vi "UHR-Fleezers Control (host) - 11.8.vi"() -> ()   [LabVIEW 2014] (continued)
        n1567 = local write "Trap Pos. FB Offset Factor"(w2207) -> ()
      }
      event "Trap Pos. FB Range", "Trap Pos. FB Gains", "Trap Pos. FB Mult Factor", "Trap Pos. FB Offset Factor", "Trap Pos FB Negate Action", "Trap Pos FB Monitor\nT1 or T2", "Differential FB?", "Negate Diff?": Value Change {
        n1568 = event-data() -> ()  [unwired: 7 out]
        n1569 = local read "Negate Diff?"() -> (w2221:bool)
        n1570 = xnode "Read/Write Control"("FPGA VI Reference In"=w2231, "error in"=w2230, "Trap Pos. FB Range"="Trap Pos. FB Range", "Trap Pos. FB Gains"="Trap Pos. FB Gains", "Trap Pos. FB Mult Factor"="Trap Pos. FB Mult Factor", "Trap Pos. FB Offset Factor"="Trap Pos. FB Offset Factor", "Trap Pos FB Negate Action"="Trap Pos FB Negate Action", "Trap Pos FB Monitor T1 or T2"="Trap Pos FB Monitor\nT1 or T2", "AI1 X Scale"="Trap Pos. AI1 X Pre-scale", "Negate Diff?"=w2221, "Diff FB Measurement?"="Differential FB?") -> ()  [unwired: 2 out]
      }
      event "Trap Pos FB SP", "Trap Pos FB SP 2", "Use SP 2": Value Change {
        n1571 = event-data() -> ()  [unwired: 7 out]
        n1572 = Select(t="Trap Pos FB SP 2", s="Use SP 2", f="Trap Pos FB SP") -> (s? t:f=w2232:fxp<+/-,16,1>)
        n1573 = xnode "Read/Write Control"("FPGA VI Reference In"=w2237, "error in"=w2236, "Trap Pos. FB SP"=w2232) -> ()  [unwired: 2 out]
      }
      event "Offset SP2 from SP1": Value Change {
        n1574 = event-data() -> ()  [unwired: 7 out]
        n1575 = local read "Trap Pos FB SP"() -> (w2240:fxp<+/-,16,1>)
        n1576 = Add(x=w2240, y="SP2 Offset") -> (x+y=w2238:fxp<+/-,16,1>)
        n1577 = property on="Trap Pos FB SP 2" class="DigNum (strict)"("Val(Sgnl)"=w2238) -> ()  [unwired: 2 in, 2 out]
        n1578 = local write "Offset SP2 from SP1"(FALSE ("Offset SP2 from SP1")) -> ()
      }
      event "Set Reading to\nSetpoint": Value Change {
        # "This is the actual PID input signal"
        n1579 = event-data() -> ()  [unwired: 7 out]
        n1580 = local write "Set Reading to\nSetpoint"(FALSE ("Set SP to Reading")) -> ()
        n1581 = xnode "Read/Write Control"("FPGA VI Reference In"=w2246, "error in"=w2245) -> ("FPGA VI Reference Out"=w2244:T19, "error out"=w2243:errorcluster, "Trap Pos FB Int-Norm Signal"=w2242:fxp<+/-,16,1>)
        n1582 = local read "Differential FB?"() -> (w2247:bool)
        n1583 = case shown="False" w2247 {
          tunnel: [w2252 w2259] -> w2249
          tunnel: w2242 -> [w2250 w2259]
          frame False {
            n1584 = local read "Trap Pos FB Monitor\nT1 or T2"() -> (w2255:bool)
            n1585 = local read "Trap X AI1 (DMA)"() -> (w2258:T13)
            n1586 = Unbundle By Name(w2258) -> ("Set 1"=w2257:fxp<+/-,16,1>, "Set 2"=w2256:fxp<+/-,16,1>)
            n1587 = Select(t=w2257, s=w2255, f=w2256) -> (s? t:f=w2254:fxp<+/-,16,1>)
            n1588 = Not(x="Set SP Using...") -> (.not. x?=w2251:bool)
            n1589 = Select(t=w2250, s=w2251, f=w2254) -> (s? t:f=w2252:fxp<+/-,16,1>)
          }
          frame True {
          }
        }
        n1590 = xnode "Read/Write Control"("FPGA VI Reference In"=w2244, "error in"=w2243, "Trap Pos. FB SP"=w2249) -> ()  [unwired: 2 out]
        n1591 = local write "Trap Pos FB SP"(w2249) -> ()
      }
      event "Trap Pos. FB Out Scale 2^n": Value Change {
        n1592 = event-data() -> ()  [unwired: 7 out]
        n1593 = Scale By Power Of 2(n="Trap Pos. FB Out Scale 2^n", x=ext 1.0) -> (x*2^n=w2260:ext)
        n1594 = property on="Trap Pos. FB Mult Factor" class="DigNum (strict)"("Val(Sgnl)"=w2260) -> ()  [unwired: 2 in, 2 out]
      }
      event "Trap Pos FB Int Count": Value Change {
        n1595 = event-data() -> ()  [unwired: 7 out]
        n1596 = xnode "Read/Write Control"("FPGA VI Reference In"=w2265, "error in"=w2264, "Trap Pos FB Int Count"="Trap Pos FB Int Count") -> ()  [unwired: 2 out]
      }
      event "Trap pos": Value Change {
        n1597 = event-data() -> ()  [unwired: 7 out]
        n1598 = case shown="True" "Trap pos" {
          frame False {
            n1599 = property on="Trap Delta Graph" class="WFGraph (strict)"("Visible"=TRUE) -> ()  [unwired: 2 in, 2 out]
            n1600 = property on="Saved trap pos" class="WFGraph (strict)"("Visible"=FALSE) -> ()  [unwired: 2 in, 2 out]
          }
          frame True {
            n1601 = property on="Saved trap pos" class="WFGraph (strict)"("Visible"=TRUE) -> ()  [unwired: 2 in, 2 out]
            n1602 = property on="Trap Delta Graph" class="WFGraph (strict)"("Visible"=FALSE) -> ()  [unwired: 2 in, 2 out]
          }
        }
      }
      event "Save user params": Value Change {
        n1603 = event-data() -> ()  [unwired: 7 out]
        n1604 = local write "Save user params"(FALSE ("Save user\nparams")) -> ()
        n1605 = call "save control values.vi"("User"="User") -> ()  [unwired: 8 in, 1 out]
        n1606 = local read "Messages"() -> (w2277:string)
        n1607 = Concatenate Strings("User: ", "User", "\r", "Parameters saved.") -> (w2272:string)
        n1608 = call "Update messages.vi"("Message to add"=w2272, "Old message string"=w2277) -> ("New message string"=w2271:string)
        n1609 = local write "Messages"(w2271) -> ()
      }
      event "Load user params": Value Change {
        n1610 = event-data() -> ()  [unwired: 7 out]
        n1611 = local write "Load user params"(FALSE ("Read user\nparams")) -> ()
        n1612 = flat-sequence {
          tunnel: [w2309] -> w2297
          tunnel: [w2308] -> w2295
          tunnel: [w2307] -> w2293
          tunnel: [w2306] -> w2291
          tunnel: [w2305] -> w2289
          tunnel: [w2304] -> w2287
          tunnel: [w2303] -> w2285
          tunnel: [w2302] -> w2283
          tunnel: [w2301] -> w2281
          tunnel: [w2300] -> w2279
          tunnel: [w2319] -> w2298
          tunnel: w2297 -> [w2319]
          tunnel: [w2318] -> w2296
          tunnel: w2295 -> [w2318]
          tunnel: [w2317] -> w2294
          tunnel: w2293 -> [w2317]
          tunnel: [w2316] -> w2292
          tunnel: w2291 -> [w2316]
          tunnel: [w2315] -> w2290
          tunnel: w2289 -> [w2315]
          tunnel: [w2314] -> w2288
          tunnel: w2287 -> [w2314]
          tunnel: [w2313] -> w2286
          tunnel: w2285 -> [w2313]
          tunnel: [w2312] -> w2284
          tunnel: w2283 -> [w2312]
          tunnel: [w2311] -> w2282
          tunnel: w2281 -> [w2311]
          tunnel: [w2310] -> w2280
          tunnel: w2279 -> [w2310]
          tunnel: w2298 -> [w2336]
          tunnel: w2296 -> [w2335]
          tunnel: w2294 -> [w2334]
          tunnel: w2292 -> [w2333]
          tunnel: w2290 -> [w2332]
          tunnel: w2288 -> [w2331]
          tunnel: w2286 -> [w2330]
          tunnel: w2284 -> [w2329]
          tunnel: w2282 -> [w2328]
          tunnel: w2280 -> [w2327]
          frame #0 {
            # "Make exceptions.\nThese will not be\nloaded."
            n1613 = local read "Green Laser ON/Interlacing"() -> (w2305:bool)
            n1614 = local read "Sample Channel\nFlow"() -> (w2304:bool)
            n1615 = local read "Trap 1 (ON/OFF)"() -> (w2309:bool)
            n1616 = local read "Trap 2 (ON/OFF)"() -> (w2308:bool)
            n1617 = local read "Trap Pos. FB ON"() -> (w2300:bool)
            n1618 = local read "Inject Pump 1"() -> (w2303:bool)
            n1619 = local read "Inject Pump 3"() -> (w2302:bool)
            n1620 = local read "Trap D (MHz)"() -> (w2301:dbl)
            n1621 = local read "Index"() -> (w2306:dbl)
            n1622 = local read "Fish"() -> (w2307:bool)
          }
          frame #1 {
            n1623 = local read "User"() -> (w2320:string)
            n1624 = call "retrieve control values.vi"("User"=w2320) -> ()  [unwired: 10 in, 1 out]
            n1625 = local read "Messages"() -> (w2326:string)
            n1626 = Concatenate Strings("User: ", w2320, "\r", "Parameters loaded.") -> (w2321:string)
            n1627 = call "Update messages.vi"("Message to add"=w2321, "Old message string"=w2326) -> ("New message string"=w2325:string)
            n1628 = local write "Messages"(w2325) -> ()
          }
          frame #2 {
            n1629 = local write "Green Laser ON/Interlacing"(w2332) -> ()
            n1630 = local write "Sample Channel\nFlow"(w2331) -> ()
            n1631 = local write "Trap 1 (ON/OFF)"(w2336) -> ()
            n1632 = local write "Trap 2 (ON/OFF)"(w2335) -> ()
            n1633 = local write "Inject Pump 1"(w2330) -> ()
            n1634 = local write "Trap Pos. FB ON"(w2327) -> ()
            n1635 = local write "Inject Pump 3"(w2329) -> ()
            n1636 = local write "Trap D (MHz)"(w2328) -> ()
            n1637 = local write "Index"(w2333) -> ()
            n1638 = local write "Fish"(w2334) -> ()
          }
        }
      }
      event "Abort wiggle": Value Change {
        n1639 = event-data() -> ()  [unwired: 7 out]
        n1640 = flat-sequence {
          tunnel: w2340 -> [w2344]
          tunnel: w2339 -> [w2343]
          tunnel: [w2342] -> w2337
          tunnel: [w2346] -> w2338
          tunnel: w2337 -> [w2346]
          frame #0 {
            n1641 = xnode "Read/Write Control"("FPGA VI Reference In"=w2344, "error in"=w2343, "Abort wiggle 1"="Abort wiggle", "Abort wiggle 2"="Abort wiggle") -> ("error out"=w2342:errorcluster)  [unwired: 1 out]
          }
          frame #1 {
            n1642 = local write "Abort wiggle"(FALSE ("Abort wiggle")) -> ()
          }
        }
      }
    }
    "error out 2" <- w1142
    n1643 = node-c288() -> ()  [unwired: 2 out]
  }
  n1644 = node-c288() -> (w96:T21)  [unwired: 4 in]
  n1645 = node-c288() -> (w110:T21)  [unwired: 4 out]
  n1646 = timed-loop "Run Scripts, including: stage motion" {
    tunnel: w101 -> [w2354]
    tunnel: w100 -> [w2355]
    tunnel: [w2355] -> w99
    tunnel: [w2354] -> w98
    timing: w96 -> [_]
    timing-out: [_] -> w95
    tunnel: w81 -> [w2353]
    tunnel: w82 -> [w2352]
    tunnel: w22 -> [w2349]
    tunnel: w21 -> [w2348]
    tunnel: w20 -> [w2350]
    tunnel: w19 -> [w2351]
    stop <- w2347 stop-if-true
    n1647 = node-c288() -> ()  [unwired: 1 in, 1 out]
    n1648 = event shown="[12] \"Force FB Script\": Value Change" {
      selector: _ -> [_ _ _ _ _ _ _ _ _ _ _ _ _ _ _ _ _ _ _ _]
      dyn-events: _ -> [_ _ _ _ _ _ _ _ _ _ _ _ _ _ _ _ _ _ _ _]
      timeout: _ -> [_ _ _ _ _ _ _ _ _ _ _ _ _ _ _ _ _ _ _ _]
      tunnel: ["Set Position" "Move to Position" _ _ "Read Harvard" _ _ _ _ _ _ "Got ADig bead" "Force FB Script" "Rupture Script" _ "Got DNA bead" "Take Stepping Data" _ "Take Detection Laser\nImage" _] -> _
      tunnel: [_ _ _ _ _ _ _ _ _ _ _ _ _ _ _ _ _ _ _ w3010] -> w2347
      tunnel: w2354 -> [w2373 w2381 w2394 w2424 _ w2471 w2511 w2592 w2623 w2757 w2783 _ w2821 _ _ _ _ _ _ _]
      tunnel: w2355 -> [w2374 w2382 w2395 w2425 _ w2472 w2512 w2593 w2624 w2758 w2784 _ w2822 _ _ _ _ _ _ _]
      tunnel: w2353 -> [_ _ _ _ w2456 _ _ _ _ _ _ _ _ _ _ _ _ _ _ _]
      tunnel: w2352 -> [_ _ _ _ w2455 _ _ _ _ _ _ _ _ _ _ _ _ _ _ _]
      tunnel: w2351 -> [_ _ _ _ _ _ _ _ _ _ _ _ _ _ _ _ _ _ _ _]
      tunnel: w2350 -> [_ _ _ _ _ _ _ _ _ _ _ _ _ _ _ _ _ _ _ _]
      tunnel: w2349 -> [_ _ _ _ _ _ _ _ _ _ _ _ _ _ _ _ _ _ _ _]
      tunnel: w2348 -> [_ _ _ _ _ _ _ _ _ _ _ _ _ _ _ _ _ _ _ _]
      event "Set Position", "Set Position 2", "Set Position 3", "Set Position 4", "Set Position 5", "Set Position 1": Value Change {
        n1649 = event-data() -> ()  [unwired: 1 in, 5 out]
        n1650 = Build Array("Set Position 1", "Set Position 2", "Set Position 3", "Set Position 4", "Set Position 5") -> (w2372:bool[])
        n1651 = Boolean Array To Number(Boolean array=w2372) -> (number=w2371:u32)
        n1652 = Logarithm Base 2(1:w2371) -> (0:w2363:dbl)
        n1653 = call "Read Stage Position.vi"("error in"=w2373, "VISA resource name in"=w2374) -> ("Current Position"=w2378:cluster{dbl, dbl, dbl}, "error out"=w2377:errorcluster)  [unwired: 2 out]
        n1654 = Decrement(x="Position") -> (x-1=w2361:dbl)
        n1655 = Greater Or Equal?(x=w2363, y=0.0) -> (x >= y?=w2364:bool)
        n1656 = Cluster To Array(cluster=w2378) -> (array=w2375:dbl[])
        n1657 = local write "Stage Control Serial Error"(w2377) -> ()
        n1658 = Select(t=w2363, s=w2364, f=w2361) -> (s? t:f=w2360:dbl)
        n1659 = Increment(x=w2360) -> (x+1=w2359:dbl)
        n1660 = Build Array (concatenate)(w2359, w2375) -> (w2358:dbl[])
        n1661 = Replace Array Subset(array="Saved Stage Positions", new element=w2358, index (row)=w2360) -> (w2376:dbl[][])  [unwired: 1 in]
        n1662 = local write "Saved Stage Positions"(w2376) -> ()
      }
      event "Move to Position": Value Change {
        n1663 = event-data() -> ()  [unwired: 1 in, 5 out]
        n1664 = flat-sequence {
          tunnel: w2382 -> [w2386]
          tunnel: w2381 -> [w2385]
          frame #0 {
            n1665 = local read "Saved Stage Positions"() -> (w2388:dbl[][])
            n1666 = local read "Position"() -> (w2387:dbl)
            n1667 = local write "Stage Moving"(TRUE ("Stage Moving")) -> ()
            n1668 = call "move to saved stage position.vi"("error in"=w2385, "Stage VISA resource name in"=w2386, "Position"=w2387, "Saved Stage Positions"=w2388) -> ("error out"=w2384:errorcluster)  [unwired: 1 out]
            n1669 = local write "Stage Control Serial Error"(w2384) -> ()
          }
          frame #1 {
            n1670 = call <vilib>:"Beep.vi"() -> ()  [unwired: 3 in, 9 out]
            n1671 = local write "Stage Moving"(FALSE ("Stage Moving")) -> ()
          }
        }
      }
      event "Move Cap. 1 (DNA Bottom)": Value Change {
        n1672 = event-data() -> ()  [unwired: 1 in, 5 out]
        n1673 = local write "Move Cap. 1 (DNA Bottom)"(FALSE ("Move Cap. 1 (DNA Right)")) -> ()
        n1674 = flat-sequence {
          tunnel: w2394 -> [w2397]
          tunnel: w2395 -> [w2398]
          tunnel: [w2398] -> w2392
          tunnel: [w2397] -> w2391
          tunnel: w2392 -> [w2400]
          tunnel: w2391 -> [w2399]
          frame #0 {
            n1675 = property on="Sample Channel\nFlow" class="Bool (strict)"("Val(Sgnl)"="Cap 1 Samp Flow ON") -> ()  [unwired: 2 in, 2 out]
          }
          frame #1 {
            n1676 = local read "Saved Stage Positions"() -> (w2410:dbl[][])
            n1677 = local write "Stage Moving"(TRUE ("Stage Moving")) -> ()
            n1678 = Array Subset(array=w2410, index (row)=0 ("index"), length (row)=1 ("length"), index (col)=1 ("index"), length (col)=3 ("length")) -> (w2407:dbl[][])
            n1679 = Reshape Array(w2407, 3 ("dimension size")) -> (w2405:dbl[])
            n1680 = Array To Cluster(array=w2405) -> (cluster=w2404:cluster{"[0]":dbl, "[1]":dbl, "[2]":dbl})
            n1681 = call "Set Stage Position.vi"("Position"=w2404, "error in"=w2399, "VISA resource name in"=w2400) -> ("error out"=w2403:errorcluster)  [unwired: 2 out]
            n1682 = local write "Stage Control Serial Error"(w2403) -> ()
          }
          frame #2 {
            n1683 = local write "Stage Moving"(FALSE ("Stage Moving")) -> ()
            n1684 = case shown="True" "Cap 1 Flow ON" {
              frame False {
              }
              frame True {
                n1685 = property on="Inject Pump 1" class="Bool (strict)"("Val(Sgnl)"=TRUE ("Value (Signaling)")) -> ()  [unwired: 2 in, 2 out]
              }
            }
            n1686 = call <vilib>:"Beep.vi"() -> ()  [unwired: 3 in, 9 out]
          }
          frame #3 {
            n1687 = property on="Sample Channel\nFlow" class="Bool (strict)"("Val(Sgnl)"=FALSE ("Value (Signaling)")) -> ()  [unwired: 2 in, 2 out]
            n1688 = local read "Cap. 2 BD T1?\n(ADig T1, DNA T2)"() -> (w2417:bool)
            n1689 = case shown="True" w2417 {
              tunnel: "Cap 1 T ON" -> [w2419 w2420]
              frame False {
                n1690 = property on="Trap 1 (ON/OFF)" class="Bool (strict)"("Val(Sgnl)"=w2419) -> ()  [unwired: 2 in, 2 out]
              }
              frame True {
                n1691 = property on="Trap 2 (ON/OFF)" class="Bool (strict)"("Val(Sgnl)"=w2420) -> ()  [unwired: 2 in, 2 out]
              }
            }
            n1692 = property on="Got DNA bead" class="Bool"("Key Focus"=TRUE) -> ()  [unwired: 2 in, 2 out]
          }
        }
      }
      event "Move Cap. 2 (ADig Top)": Value Change {
        n1693 = event-data() -> ()  [unwired: 1 in, 5 out]
        n1694 = local write "Move Cap. 2 (ADig Top)"(FALSE ("Move Cap. 2 (ADig Left)")) -> ()
        n1695 = flat-sequence {
          tunnel: w2424 -> [w2427]
          tunnel: w2425 -> [w2428]
          tunnel: [w2428] -> w2422
          tunnel: [w2427] -> w2421
          tunnel: w2422 -> [w2431]
          tunnel: w2421 -> [w2430]
          frame #0 {
            n1696 = property on="Sample Channel\nFlow" class="Bool (strict)"("Val(Sgnl)"="Cap 2 Samp Flow ON") -> ()  [unwired: 2 in, 2 out]
          }
          frame #1 {
            w2429 = FALSE ("Value (Signaling)")
            n1697 = local read "Saved Stage Positions"() -> (w2441:dbl[][])
            n1698 = local write "Stage Moving"(TRUE ("Stage Moving")) -> ()
            n1699 = Array Subset(array=w2441, index (row)=1 ("index"), length (row)=1 ("length"), index (col)=1 ("index"), length (col)=3 ("length")) -> (w2438:dbl[][])
            n1700 = Reshape Array(w2438, 3 ("dimension size")) -> (w2436:dbl[])
            n1701 = property on="Trap 1 (ON/OFF)" class="Bool (strict)"("Val(Sgnl)"=w2429) -> ()  [unwired: 2 in, 2 out]
            n1702 = property on="Trap 1 (ON/OFF)" class="Bool (strict)"("Val(Sgnl)"=w2429) -> ()  [unwired: 2 in, 2 out]
            n1703 = Array To Cluster(array=w2436) -> (cluster=w2435:cluster{"[0]":dbl, "[1]":dbl, "[2]":dbl})
            n1704 = call "Set Stage Position.vi"("Position"=w2435, "error in"=w2430, "VISA resource name in"=w2431) -> ("error out"=w2434:errorcluster)  [unwired: 2 out]
            n1705 = local write "Stage Control Serial Error"(w2434) -> ()
          }
          frame #2 {
            n1706 = local write "Stage Moving"(FALSE ("Stage Moving")) -> ()
            n1707 = call <vilib>:"Beep.vi"() -> ()  [unwired: 3 in, 9 out]
            n1708 = case shown="True" "Cap 2 Flow ON" {
              frame False {
              }
              frame True {
                n1709 = property on="Inject Pump 3" class="Bool (strict)"("Val(Sgnl)"=TRUE ("Value (Signaling)")) -> ()  [unwired: 2 in, 2 out]
              }
            }
          }
          frame #3 {
            n1710 = local read "Cal @ (MHz)"() -> (w2447:dbl)
            n1711 = property on="Sample Channel\nFlow" class="Bool (strict)"("Val(Sgnl)"=FALSE ("Value (Signaling)")) -> ()  [unwired: 2 in, 2 out]
            n1712 = case shown="False" "Cap. 2 BD T1?\n(ADig T1, DNA T2)" {
              tunnel: "Cap 2 T ON" -> [w2452 w2453]
              frame False {
                n1713 = property on="Trap 2 (ON/OFF)" class="Bool (strict)"("Val(Sgnl)"=w2452) -> ()  [unwired: 2 in, 2 out]
              }
              frame True {
                n1714 = property on="Trap 1 (ON/OFF)" class="Bool (strict)"("Val(Sgnl)"=w2453) -> ()  [unwired: 2 in, 2 out]
              }
            }
            n1715 = property on="Got ADig bead" class="Bool"("Key Focus"=TRUE) -> ()  [unwired: 2 in, 2 out]
            n1716 = local write "Target"("Target\nON?") -> ()
            n1717 = property on="Trap D (MHz)" class="DigNum (strict)"("Val(Sgnl)"=w2447) -> ()  [unwired: 2 in, 2 out]
          }
        }
      }
      event "Read Harvard": Value Change {
        n1718 = event-data() -> ()  [unwired: 1 in, 5 out]
        n1719 = Concatenate Strings("write buffer", "\r") -> (w2458:string)
        n1720 = VISA Write(VISA resource name=w2456, write buffer=w2458, error in (no error)=w2455) -> (VISA resource name out=w2467:refnum<visa-resource-name>, error out=w2466:errorcluster)  [unwired: 1 out]
        n1721 = stacked-sequence {
          tunnel: [w2470] -> w2465
          tunnel: w2467 -> [w2470]
          tunnel: w2466 -> [w2469]
          tunnel: [w2469] -> w2460
          frame #0 {
            n1722 = Wait (ms)(milliseconds to wait=50) -> ()  [unwired: 1 out]
          }
        }
        n1723 = property class="Instr"(reference=w2465, error in=w2460) -> (reference out=w2464:refnum<visa-resource-name>, error out=w2462:errorcluster, "Serial Settings:Number of Bytes at Serial Port"=w2463:u32)
        "Serial Settings:Number of Bytes at Serial Port" <- w2463
        n1724 = VISA Read(VISA resource name=w2464, byte count=w2463, error in (no error)=w2462) -> (read buffer=w2461:string)  [unwired: 3 out]
        "read buffer" <- w2461
        n1725 = Fract/Exp String To Number(string=w2461) -> ()  [unwired: 5 out]
      }
      event "+z", "-z": Value Change {
        n1726 = event-data() -> ()  [unwired: 1 in, 5 out]
        n1727 = flat-sequence {
          tunnel: w2471 -> [w2493]
          tunnel: w2472 -> [w2473]
          frame #0 {
            n1728 = call "Read Stage Position.vi"("error in"=w2493, "VISA resource name in"=w2473) -> ("Current Position"=w2478:cluster{dbl, dbl, dbl}, "error out"=w2491:errorcluster, "VISA resource name out"=w2492:refnum<visa-resource-name>)  [unwired: 1 out]
            n1729 = local read "Saved Stage Positions"() -> (w2502:dbl[][])
            n1730 = Divide(x="z nudge increment (um)", y=1000.0) -> (x/y=w2490:dbl)
            n1731 = Boolean To (0,1)(Boolean="+z") -> (0, 1=w2482:i16)
            n1732 = Boolean To (0,1)(Boolean="-z") -> (0, 1=w2483:i16)
            n1733 = Array Subset(array=w2502, index (row)=1 ("index"), length (row)=1 ("length"), index (col)=1 ("index"), length (col)=3 ("length")) -> (w2499:dbl[][])
            n1734 = Multiply(x=w2482, y=w2490) -> (x*y=w2486:dbl)
            n1735 = Multiply(x=w2483, y=w2490) -> (x*y=w2484:dbl)
            n1736 = Unbundle(w2478) -> (w2476:dbl, w2475:dbl, w2479:dbl)
            n1737 = Negate(x=w2484) -> (-x=w2485:dbl)
            n1738 = Reshape Array(w2499, 3 ("dimension size")) -> (w2497:dbl[])
            n1739 = Add(x=w2486, y=w2485) -> (x+y=w2487:dbl)
            n1740 = Array To Cluster(array=w2497) -> ()  [unwired: 1 out]
            n1741 = Add(x=w2487, y=w2479) -> (x+y=w2477:dbl)
            n1742 = Bundle(cluster=w2478, w2476, w2475, w2477) -> (w2474:cluster{dbl, dbl, dbl})
            n1743 = call "Set Stage Position.vi"("Position"=w2474, "error in"=w2491, "VISA resource name in"=w2492) -> ("error out"=w2496:errorcluster)  [unwired: 2 out]
            n1744 = local write "Stage Moving"(TRUE ("Stage Moving")) -> ()
            n1745 = local write "Stage Control Serial Error"(w2496) -> ()
          }
          frame #1 {
            n1746 = local write "Stage Moving"(FALSE ("Stage Moving")) -> ()
            n1747 = call <vilib>:"Beep.vi"() -> ()  [unwired: 3 in, 9 out]
          }
        }
      }
      event "Cal/Data Acq. Spot": Value Change {
        n1748 = event-data() -> ()  [unwired: 1 in, 5 out]
        n1749 = flat-sequence {
          tunnel: w2511 -> [w2515]
          tunnel: w2512 -> [w2516]
          tunnel: [w2516] -> w2508
          tunnel: [w2515] -> w2507
          tunnel: w2508 -> [w2521]
          tunnel: w2507 -> [w2520]
          tunnel: ["Cal @ (MHz)"] -> w2505
          tunnel: [w2525] -> w2509
          tunnel: w2505 -> [w2525]
          tunnel: w2509 -> [w2534]
          tunnel: ["W/ Offset 1"] -> w2506
          tunnel: w2509 -> [w2555]
          tunnel: w2506 -> [w2553]
          frame #0 {
            n1750 = property on="Sample Channel\nFlow" class="Bool (strict)"("Val(Sgnl)"="Daq spot flow on") -> ()  [unwired: 2 in, 2 out]
            n1751 = Wait (ms)(milliseconds to wait=u32 250) -> ()  [unwired: 1 out]
          }
          frame #1 {
            n1752 = local read "Saved Stage Positions"() -> (w2518:dbl[][])
            n1753 = property on="Trap D (MHz)" class="DigNum (strict)"("Val(Sgnl)"="Cal @ (MHz)") -> ()  [unwired: 2 in, 2 out]
            n1754 = local write "Stage Moving"(TRUE ("Stage Moving")) -> ()
            n1755 = call "move to saved stage position.vi"("error in"=w2520, "Stage VISA resource name in"=w2521, "Position"="Cal Stage Position", "Saved Stage Positions"=w2518) -> ("error out"=w2519:errorcluster)  [unwired: 1 out]
            n1756 = local write "Stage Control Serial Error"(w2519) -> ()
          }
          frame #2 {
            n1757 = local write "Stage Moving"(FALSE ("Stage Moving")) -> ()
            n1758 = property on="Sample Channel\nFlow" class="Bool (strict)"("Val(Sgnl)"="Flow ON\nduring cal?") -> ()  [unwired: 2 in, 2 out]
            n1759 = call <vilib>:"Beep.vi"() -> ()  [unwired: 3 in, 9 out]
          }
          frame #3 {
            n1760 = Wait (ms)(milliseconds to wait=u32 1000) -> ()  [unwired: 1 out]
          }
          frame #4 {
            n1761 = property on="Save Calibration" class="Bool (strict)"("Val(Sgnl)"=TRUE ("Value (Signaling)")) -> ()  [unwired: 2 in, 2 out]
          }
          frame #5 {
            n1762 = Wait (ms)(milliseconds to wait=u32 2000) -> ()  [unwired: 1 out]
          }
          frame #6 {
            # "Check to see if \nsaving done"
            n1763 = while {
              stop <- w2530 stop-if-true
              n1764 = local read "Saving..."() -> (w2531:bool)
              n1765 = Wait (ms)(milliseconds to wait=u32 100) -> ()  [unwired: 1 out]
              n1766 = Not(x=w2531) -> (.not. x?=w2530:bool)
            }
          }
          frame #7 {
            n1767 = case shown="True" "W/ Offset 1" {
              tunnel: w2534 -> [_ w2535]
              frame False {
              }
              frame True {
                n1768 = stacked-sequence {
                  tunnel: w2535 -> [_ _ _ _ _ _ _ w2552]
                  frame #0 {
                    n1769 = property on="Trap D (MHz)" class="DigNum (strict)"("Val(Sgnl)"="Offset 1 Start (MHz)") -> ()  [unwired: 2 in, 2 out]
                    n1770 = Replace Array Subset(array=u32[] [0] ("Index Values"), new element="Offset 1 Set", index=0) -> (w2536:u32[])
                    n1771 = property on="Saved AOD Raster Scan Parameter Sets" class="Arr (strict)"("Index Values"=w2536) -> ()  [unwired: 2 in, 2 out]
                  }
                  frame #1 {
                    n1772 = Wait (ms)(milliseconds to wait=u32 200) -> ()  [unwired: 1 out]
                  }
                  frame #2 {
                    n1773 = property on="Load parameters" class="Bool (strict)"("Val(Sgnl)"=TRUE ("Value (Signaling)")) -> ()  [unwired: 2 in, 2 out]
                  }
                  frame #3 {
                    n1774 = Wait (ms)(milliseconds to wait=u32 200) -> ()  [unwired: 1 out]
                  }
                  frame #4 {
                    n1775 = property on="Trap Raster Scan" class="Bool (strict)"("Val(Sgnl)"=TRUE ("Value (Signaling)")) -> ()  [unwired: 2 in, 2 out]
                  }
                  frame #5 {
                    n1776 = Wait (ms)(milliseconds to wait=u32 2000) -> ()  [unwired: 1 out]
                  }
                  frame #6 {
                    n1777 = while {
                      stop <- w2549 stop-if-true
                      n1778 = local read "Raster Scanning..."() -> (w2551:bool)
                      n1779 = local read "Saving..."() -> (w2547:bool)
                      n1780 = Wait (ms)(milliseconds to wait=u32 100) -> ()  [unwired: 1 out]
                      n1781 = Not(x=w2547) -> (.not. x?=w2546:bool)
                      n1782 = Not(x=w2551) -> (.not. x?=w2548:bool)
                      n1783 = And(x=w2548, y=w2546) -> (x .and. y?=w2549:bool)
                    }
                  }
                  frame #7 {
                    n1784 = property on="Trap D (MHz)" class="DigNum (strict)"("Val(Sgnl)"=w2552) -> ()  [unwired: 2 in, 2 out]
                  }
                }
              }
            }
          }
          frame #8 {
            n1785 = local read "Save ave N"() -> (w2554:dbl)
            n1786 = case shown="False" "W/ Offset 2" {
              tunnel: w2555 -> [_ w2562]
              tunnel: w2554 -> [_ w2561]
              tunnel: w2553 -> [w2557 _]
              frame False {
                n1787 = case shown="False" w2557 {
                  frame False {
                    n1788 = Multiply(x="Cal read wait (s)", y=u32 1000 ("milliseconds to wait")) -> (x*y=w2559:u32)
                    n1789 = Wait (ms)(milliseconds to wait=w2559) -> ()  [unwired: 1 out]
                  }
                  frame True {
                  }
                }
              }
              frame True {
                n1790 = stacked-sequence {
                  tunnel: w2562 -> [_ _ _ _ _ _ _ _ _ w2583 _ _]
                  tunnel: w2561 -> [_ _ _ _ _ _ _ _ _ w2581 _ _]
                  frame #0 {
                    n1791 = property on="Save ave N" class="DigNum (strict)"("Val(Sgnl)"=1.0 ("Value (Signaling)")) -> ()  [unwired: 2 in, 2 out]
                  }
                  frame #1 {
                    n1792 = Wait (ms)(milliseconds to wait=u32 500) -> ()  [unwired: 1 out]
                  }
                  frame #2 {
                    n1793 = property on="Trap D (MHz)" class="DigNum (strict)"("Val(Sgnl)"="Offset 2 Start (MHz)") -> ()  [unwired: 2 in, 2 out]
                    n1794 = Replace Array Subset(array=u32[] [0] ("Index Values"), new element="Offset 2 Set", index=0) -> (w2567:u32[])
                    n1795 = property on="Saved AOD Raster Scan Parameter Sets" class="Arr (strict)"("Index Values"=w2567) -> ()  [unwired: 2 in, 2 out]
                  }
                  frame #3 {
                    n1796 = Wait (ms)(milliseconds to wait=u32 500) -> ()  [unwired: 1 out]
                  }
                  frame #4 {
                    n1797 = property on="Load parameters" class="Bool (strict)"("Val(Sgnl)"=TRUE ("Value (Signaling)")) -> ()  [unwired: 2 in, 2 out]
                  }
                  frame #5 {
                    n1798 = Wait (ms)(milliseconds to wait=u32 500) -> ()  [unwired: 1 out]
                  }
                  frame #6 {
                    n1799 = property on="Trap Raster Scan" class="Bool (strict)"("Val(Sgnl)"=TRUE ("Value (Signaling)")) -> ()  [unwired: 2 in, 2 out]
                  }
                  frame #7 {
                    n1800 = Wait (ms)(milliseconds to wait=u32 2000) -> ()  [unwired: 1 out]
                  }
                  frame #8 {
                    n1801 = while {
                      stop <- w2576 stop-if-true
                      n1802 = local read "Raster Scanning..."() -> (w2579:bool)
                      n1803 = local read "Saving..."() -> (w2577:bool)
                      n1804 = Wait (ms)(milliseconds to wait=u32 100) -> ()  [unwired: 1 out]
                      n1805 = Not(x=w2577) -> (.not. x?=w2575:bool)
                      n1806 = Not(x=w2579) -> (.not. x?=w2578:bool)
                      n1807 = And(x=w2578, y=w2575) -> (x .and. y?=w2576:bool)
                    }
                  }
                  frame #9 {
                    n1808 = property on="Trap D (MHz)" class="DigNum (strict)"("Val(Sgnl)"=w2583) -> ()  [unwired: 2 in, 2 out]
                    n1809 = property on="Saved AOD Raster Scan Parameter Sets" class="Arr (strict)"("Index Values"=u32[] [0]) -> ()  [unwired: 2 in, 2 out]
                    n1810 = property on="Save ave N" class="DigNum (strict)"("Val(Sgnl)"=w2581) -> ()  [unwired: 2 in, 2 out]
                  }
                  frame #10 {
                    n1811 = Wait (ms)(milliseconds to wait=u32 500) -> ()  [unwired: 1 out]
                  }
                  frame #11 {
                    n1812 = property on="Load parameters" class="Bool (strict)"("Val(Sgnl)"=TRUE ("Value (Signaling)")) -> ()  [unwired: 2 in, 2 out]
                  }
                }
              }
            }
          }
          frame #9 {
            n1813 = property on="Read Cal" class="Bool (strict)"("Val(Sgnl)"=TRUE ("Value (Signaling)")) -> ()  [unwired: 2 in, 2 out]
          }
          frame #10 {
            n1814 = Wait (ms)(milliseconds to wait=u32 1000) -> ()  [unwired: 1 out]
          }
          frame #11 {
            n1815 = property on="Fish" class="Bool (strict)"("Val(Sgnl)"=TRUE ("Value (Signaling)")) -> ()  [unwired: 2 in, 2 out]
          }
        }
        n1816 = local write "Cal/Data Acq. Spot"(FALSE ("Cal/Data Acq. Spot")) -> ()
      }
      event "Dump Beads": Value Change {
        n1817 = event-data() -> ()  [unwired: 1 in, 5 out]
        n1818 = flat-sequence {
          tunnel: ["Dump spot flow on?"] -> w2589
          tunnel: [w2601] -> w2590
          tunnel: w2589 -> [w2601]
          tunnel: w2593 -> [w2606]
          tunnel: w2592 -> [w2605]
          tunnel: [w2603] -> w2591
          tunnel: w2590 -> [w2603]
          tunnel: w2591 -> [w2617]
          frame #0 {
            w2594 = FALSE ("Value (Signaling)")
            n1819 = local read "Saving..."() -> (w2596:bool)
            n1820 = local write "Dump Beads"(FALSE ("Dump Beads")) -> ()
            n1821 = property on="Inject Pump 3" class="Bool (strict)"("Val(Sgnl)"=w2594) -> ()  [unwired: 2 in, 2 out]
            n1822 = property on="Inject Pump 1" class="Bool (strict)"("Val(Sgnl)"=w2594) -> ()  [unwired: 2 in, 2 out]
            n1823 = local write "Stop Saving"(w2596) -> ()
            n1824 = local write "Fish"(w2594) -> ()
          }
          frame #1 {
            w2597 = TRUE
            w2598 = FALSE ("Fl. Triggered...")
            n1825 = case shown="True" "Dump spot flow on?" {
              frame False {
              }
              frame True {
                n1826 = property on="Sample Channel\nFlow" class="Bool (strict)"("Val(Sgnl)"=TRUE ("Stage Moving")) -> ()  [unwired: 2 in, 2 out]
              }
            }
            n1827 = local write "Fl. Triggered..."(w2598) -> ()
            n1828 = local write "Tether"(w2598) -> ()
            n1829 = local write "Multiple tether"(w2598) -> ()
            n1830 = local write "Good tether"(w2598) -> ()
            n1831 = property on="Green Laser ON/Interlacing" class="Bool (strict)"("Val(Sgnl)"=w2598) -> ()  [unwired: 2 in, 2 out]
            n1832 = property on="Trap Pos. FB ON" class="Bool (strict)"("Val(Sgnl)"=w2598) -> ()  [unwired: 2 in, 2 out]
            n1833 = property on="Trap Trig. Fl." class="Bool (strict)"("Val(Sgnl)"=w2598) -> ()  [unwired: 2 in, 2 out]
            n1834 = local write "Bad fit"(w2598) -> ()
            n1835 = local write "Hysteresis"(w2598) -> ()
            n1836 = property on="Fl. Triggered..." class="Bool (strict)"("Val(Sgnl)"=w2598) -> ()  [unwired: 2 in, 2 out]
            n1837 = local write "Restart DMA? (AOD)"(w2597) -> ()
            n1838 = local write "Save scans"(w2597) -> ()
            n1839 = property on="Dip for Protein" class="Bool (strict)"("Val(Sgnl)"=w2598) -> ()  [unwired: 2 in, 2 out]
            n1840 = property on="Pause dwell" class="Bool (strict)"("Val(Sgnl)"=w2598) -> ()  [unwired: 2 in, 2 out]
          }
          frame #2 {
            n1841 = property on="Trap Pos. FB Offset Factor" class="DigNum (strict)"("Val(Sgnl)"=i64 0 ("Value (Signaling)")) -> ()  [unwired: 2 in, 2 out]
          }
          frame #3 {
            n1842 = local read "Saved Stage Positions"() -> (w2607:dbl[][])
            n1843 = Array Subset(array=w2607, index (row)=3 ("index"), length (row)=1 ("length"), index (col)=1 ("index"), length (col)=3 ("length")) -> (w2612:dbl[][])
            n1844 = local write "Stage Moving"(TRUE ("Stage Moving")) -> ()
            n1845 = Reshape Array(w2612, 3 ("dimension size")) -> (w2610:dbl[])
            n1846 = Array To Cluster(array=w2610) -> (cluster=w2609:cluster{"[0]":dbl, "[1]":dbl, "[2]":dbl})
            n1847 = call "Set Stage Position.vi"("Position"=w2609, "error in"=w2605, "VISA resource name in"=w2606) -> ()  [unwired: 3 out]
          }
          frame #4 {
            w2618 = FALSE ("Value (Signaling)")
            n1848 = case shown="True" w2617 {
              frame False {
              }
              frame True {
                n1849 = property on="Sample Channel\nFlow" class="Bool (strict)"("Val(Sgnl)"=FALSE ("Stage Moving")) -> ()  [unwired: 2 in, 2 out]
              }
            }
            n1850 = property on="Trap 1 (ON/OFF)" class="Bool (strict)"("Val(Sgnl)"=w2618) -> ()  [unwired: 2 in, 2 out]
            n1851 = property on="Trap 2 (ON/OFF)" class="Bool (strict)"("Val(Sgnl)"=w2618) -> ()  [unwired: 2 in, 2 out]
            n1852 = call <vilib>:"Beep.vi"() -> ()  [unwired: 3 in, 9 out]
            n1853 = local write "Fish"(FALSE ("Fish for Tether")) -> ()
          }
          frame #5 {
            n1854 = property on="Move Cap. 2 (ADig Top)" class="Bool (strict)"("Val(Sgnl)"=TRUE ("Value (Signaling)")) -> ()  [unwired: 2 in, 2 out]
            n1855 = property on="Tab Control" class="TabCtl (strict)"("Val(Sgnl)"=T4."Status" ("Value (Signaling)")) -> ()  [unwired: 2 in, 2 out]
          }
        }
      }
      event "Dip for Protein": Value Change {
        n1856 = event-data() -> ()  [unwired: 1 in, 5 out]
        n1857 = case shown="True" "Dip for Protein" {
          tunnel: w2624 -> [_ w2626]
          tunnel: w2623 -> [_ w2625]
          frame False {
          }
          frame True {
            n1858 = while {
              tunnel: w2626 -> [w2637]
              tunnel: w2625 -> [w2636]
              i -> [w2632]
              stop <- w2627 stop-if-true
              n1859 = Increment(x=w2632) -> (x+1=→"Dip #":i32)
              n1860 = flat-sequence {
                tunnel: w2636 -> [w2648]
                tunnel: w2637 -> [w2649]
                tunnel: [w2649] -> w2641
                tunnel: [w2648] -> w2640
                tunnel: [w2642] -> w2628
                tunnel: [w2654] -> w2635
                tunnel: [w2655] -> w2634
                tunnel: w2641 -> [w2656]
                tunnel: w2640 -> [w2657]
                tunnel: [w2652] -> w2629
                tunnel: w2628 -> [w2652]
                tunnel: [w2665] -> w2639
                tunnel: w2635 -> [w2665]
                tunnel: [w2664] -> w2638
                tunnel: w2634 -> [w2664]
                tunnel: [w2661] -> w2633
                tunnel: [w2660] -> w2630
                tunnel: w2629 -> [w2660]
                tunnel: w2638 -> [w2685]
                tunnel: w2639 -> [w2686]
                tunnel: w2633 -> [w2687]
                tunnel: w2630 -> [w2684]
                tunnel: [w2746] -> w2627
                frame #0 {
                  n1861 = local read "Trap Pos. FB ON"() -> (w2642:bool)
                  n1862 = Compound Arithmetic op=AND("Flow ON\nduring dip?", "FB OFF when \nflow ON", w2642) -> (w2643:bool)
                  n1863 = case shown="True" "Move trap \nbefore dip move?" {
                    frame False {
                    }
                    frame True {
                      n1864 = property on="Trap D (MHz)" class="DigNum (strict)"("Val(Sgnl)"="Dipping D (MHz)") -> ()  [unwired: 2 in, 2 out]
                    }
                  }
                  n1865 = property on="Green Laser ON/Interlacing" class="Bool (strict)"("Val(Sgnl)"="Green ON\nbefore dip?") -> ()  [unwired: 2 in, 2 out]
                  n1866 = property on="Sample Channel\nFlow" class="Bool (strict)"("Val(Sgnl)"="Flow ON\nduring dip?") -> ()  [unwired: 2 in, 2 out]
                  n1867 = case shown="True" w2643 {
                    frame False {
                    }
                    frame True {
                      n1868 = property on="Trap Pos. FB ON" class="Bool (strict)"("Val(Sgnl)"=FALSE ("Value (Signaling)")) -> ()  [unwired: 2 in, 2 out]
                    }
                  }
                }
                frame #1 {
                  n1869 = local read "Saved Stage Positions"() -> (w2659:dbl[][])
                  n1870 = local write "Cancel dwell"(FALSE ("Cancel dwell")) -> ()
                  n1871 = call "move to saved stage position.vi"("error in"=w2657, "Stage VISA resource name in"=w2656, "Position"="Dip Stage \nPosition", "Saved Stage Positions"=w2659) -> ("VISA resource name out"=w2654:refnum<visa-resource-name>, "error out"=w2655:errorcluster)
                }
                frame #2 {
                  n1872 = node-c288() -> (w2663:T21)  [unwired: 4 in]
                  n1873 = timed-loop {
                    timing: w2663 -> [_]
                    timing-out: [_] -> w2662
                    tunnel: [w2669] -> w2661
                    i -> [w2666]
                    stop <- w2670 stop-if-true
                    n1874 = node-c288() -> ()  [unwired: 1 in, 1 out]
                    n1875 = Greater Or Equal?(x=w2666, y="Dip Duration (s)") -> (x >= y?=w2678:bool)
                    n1876 = local read "Dip for Protein"() -> (w2671:bool)
                    n1877 = local read "Dump Beads"() -> (w2668:bool)
                    n1878 = local read "Cancel dwell"() -> (w2677:bool)
                    n1879 = local read "Pause dwell"() -> (w2674:bool)
                    n1880 = Not(x=w2671) -> (.not. x?=w2676:bool)
                    n1881 = Compound Arithmetic op=OR(w2677, w2678, w2676) -> (w2675:bool)
                    n1882 = Select(t=FALSE, s=w2674, f=w2675) -> (s? t:f=w2672:bool)
                    n1883 = Not(x=w2668) -> (.not. x?=w2667:bool)
                    n1884 = node-c288() -> ()  [unwired: 1 in, 1 out]
                    n1885 = And(x=w2671, y=w2667) -> (x .and. y?=w2669:bool)
                    n1886 = Or(x=w2672, y=w2668) -> (x .or. y?=w2670:bool)
                    "Dip Time (s)" <- w2666
                  }
                  n1887 = node-c288(w2662) -> ()  [unwired: 1 out]
                }
                frame #3 {
                  n1888 = case shown="True" w2687 {
                    tunnel: w2686 -> [_ w2692]
                    tunnel: w2685 -> [_ w2691]
                    tunnel: w2684 -> [_ w2688]
                    frame False {
                    }
                    frame True {
                      n1889 = flat-sequence {
                        tunnel: w2691 -> [w2696]
                        tunnel: w2692 -> [w2697]
                        tunnel: [w2697] -> w2690
                        tunnel: [w2696] -> w2689
                        tunnel: w2688 -> [w2693]
                        tunnel: w2690 -> [w2707]
                        tunnel: w2689 -> [w2706]
                        tunnel: w2688 -> [w2715]
                        frame #0 {
                          n1890 = local read "Sample Channel\nFlow"() -> (w2695:bool)
                          n1891 = case shown="True" w2695 {
                            tunnel: "Flow ON \nduring return\nfrom dip?" -> [w2698 w2701]
                            tunnel: w2693 -> [_ w2700]
                            frame False {
                              n1892 = case shown="True" w2698 {
                                frame False {
                                }
                                frame True {
                                n1893 = property on="Sample Channel\nFlow" class="Bool (strict)"("Val(Sgnl)"=TRUE ("Value (Signaling)")) -> ()  [unwired: 2 in, 2 out]
                                }
                              }
                            }
                            frame True {
                              n1894 = case shown="False" w2701 {
                                tunnel: w2700 -> [w2702 _]
                                frame False {
                                n1895 = property on="Trap Pos. FB ON" class="Bool (strict)"("Val(Sgnl)"=w2702) -> ()  [unwired: 2 in, 2 out]
                                n1896 = property on="Sample Channel\nFlow" class="Bool (strict)"("Val(Sgnl)"=FALSE ("Value (Signaling)")) -> ()  [unwired: 2 in, 2 out]
                                }
                                frame True {
                                }
                              }
                            }
                          }
                        }
                        frame #1 {
                          # "For turning on green laser before stage reaches lower spot"
                          n1897 = case shown="True" "Green ON\nafter start\nreturn?" {
                            frame False {
                            }
                            frame True {
                              n1898 = flat-sequence {
                                frame #0 {
                                n1899 = Multiply(x="Green delay after \nstart return (s)", y=1000.0) -> (x*y=w2712:dbl)
                                n1900 = Wait (ms)(milliseconds to wait=w2712) -> ()  [unwired: 1 out]
                                }
                                frame #1 {
                                n1901 = property on="Green Laser ON/Interlacing" class="Bool (strict)"("Val(Sgnl)"=TRUE ("Value (Signaling)")) -> ()  [unwired: 2 in, 2 out]
                                }
                              }
                            }
                          }
                          n1902 = local read "Saved Stage Positions"() -> (w2710:dbl[][])
                          n1903 = local write "Cancel dwell"(FALSE ("Cancel dwell")) -> ()
                          n1904 = call "move to saved stage position.vi"("error in"=w2706, "Stage VISA resource name in"=w2707, "Position"="Return Stage \nPosition", "Saved Stage Positions"=w2710) -> ("error out"=w2708:errorcluster)  [unwired: 1 out]
                          n1905 = local write "Stage Control Serial Error"(w2708) -> ()
                        }
                        frame #2 {
                          n1906 = property on="Trap Pos. FB ON" class="Bool (strict)"("Val(Sgnl)"=w2715) -> ()  [unwired: 2 in, 2 out]
                          n1907 = case shown="True" "Green ON \nafter return?" {
                            frame False {
                            }
                            frame True {
                              n1908 = property on="Green Laser ON/Interlacing" class="Bool (strict)"("Val(Sgnl)"=TRUE ("Value (Signaling)")) -> ()  [unwired: 2 in, 2 out]
                            }
                          }
                          n1909 = case shown="True" "Move trap after return?" {
                            frame False {
                            }
                            frame True {
                              n1910 = property on="Trap D (MHz)" class="DigNum (strict)"("Val(Sgnl)"="Dip Trap D 2 (MHz)") -> ()  [unwired: 2 in, 2 out]
                            }
                          }
                          n1911 = case shown="True" "Save data after return?" {
                            frame False {
                            }
                            frame True {
                              n1912 = property on="Start Saving" class="Bool (strict)"("Val(Sgnl)"=TRUE ("Value (Signaling)")) -> ()  [unwired: 2 in, 2 out]
                            }
                          }
                          n1913 = property on="Sample Channel\nFlow" class="Bool (strict)"("Val(Sgnl)"="Flow ON\nduring daq?") -> ()  [unwired: 2 in, 2 out]
                        }
                        frame #3 {
                          n1914 = node-c288() -> (w2724:T21)  [unwired: 4 in]
                          n1915 = timed-loop {
                            timing: w2724 -> [_]
                            timing-out: [_] -> w2723
                            i -> [w2725]
                            stop <- w2727 stop-if-true
                            n1916 = node-c288() -> ()  [unwired: 1 in, 1 out]
                            n1917 = local read "Dump Beads"() -> (w2726:bool)
                            n1918 = Greater Or Equal?(x=w2725, y="Dwell Duration (s)") -> (x >= y?=w2732:bool)
                            n1919 = local read "Dip for Protein"() -> (w2729:bool)
                            n1920 = Not(x=w2729) -> (.not. x?=w2728:bool)
                            n1921 = Compound Arithmetic op=OR(w2732, "Cancel dwell", w2728) -> (w2731:bool)
                            n1922 = node-c288() -> ()  [unwired: 1 in, 1 out]
                            n1923 = Select(t=FALSE, s="Pause dwell", f=w2731) -> (s? t:f=w2734:bool)
                            n1924 = Or(x=w2734, y=w2726) -> (x .or. y?=w2727:bool)
                            "Dwell Time (s)" <- w2725
                          }
                          n1925 = node-c288(w2723) -> ()  [unwired: 1 out]
                        }
                      }
                    }
                  }
                }
                frame #4 {
                  n1926 = local read "Dip for Protein"() -> (w2743:bool)
                  n1927 = local read "Tether"() -> (w2742:bool)
                  n1928 = local read "Dump Beads"() -> (w2744:bool)
                  n1929 = local write "Cancel dwell"(FALSE ("Cancel dwell")) -> ()
                  n1930 = Not(x=w2742) -> (.not. x?=w2741:bool)
                  n1931 = Not(x=w2743) -> (.not. x?=w2747:bool)
                  n1932 = Not(x="Cont. Repeat Dipping?") -> (.not. x?=w2749:bool)
                  n1933 = Compound Arithmetic op=OR(w2741, w2747, w2749, w2744) -> (w2746:bool)
                }
              }
            }
          }
        }
      }
      event "Profile": Value Change {
        n1934 = event-data() -> ()  [unwired: 1 in, 5 out]
        n1935 = flat-sequence {
          tunnel: w2758 -> [w2761]
          tunnel: w2757 -> [w2769]
          tunnel: [w2763] -> w2756
          tunnel: [w2762] -> w2755
          tunnel: [w2760] -> w2753
          tunnel: [w2759] -> w2750
          tunnel: w2756 -> [w2776]
          tunnel: w2755 -> [w2775]
          tunnel: [w2773] -> w2754
          tunnel: w2753 -> [w2774]
          tunnel: [w2772] -> w2752
          tunnel: [w2771] -> w2751
          tunnel: w2750 -> [w2771]
          tunnel: w2754 -> [w2780]
          tunnel: w2752 -> [w2779]
          tunnel: w2751 -> [w2778]
          frame #0 {
            n1936 = call "Read Stage Position.vi"("error in"=w2769, "VISA resource name in"=w2761) -> ("Current Position"=w2759:cluster{dbl, dbl, dbl}, "error out"=w2762:errorcluster, "VISA resource name out"=w2760:refnum<visa-resource-name>)  [unwired: 1 out]
            "Current Position" <- w2759
            n1937 = local write "Stage Control Serial Error"(w2762) -> ()
            n1938 = Unbundle(w2759) -> (w2766:dbl, w2768:dbl, w2764:dbl)
            n1939 = Add(x=w2768, y="Y change (mm)") -> (x+y=w2765:dbl)
            n1940 = Bundle(w2766, w2765, w2764) -> (w2763:cluster{dbl, dbl, dbl})  [unwired: 1 in]
          }
          frame #1 {
            # "move to new position and start saving"
            n1941 = local write "Stage Moving"(TRUE ("Stage Moving")) -> ()
            n1942 = local write "Start Saving"(TRUE ("Start Saving")) -> ()
            n1943 = call "Set Stage Position.vi"("Position"=w2776, "error in"=w2775, "VISA resource name in"=w2774) -> ("error out"=w2772:errorcluster, "VISA resource name out"=w2773:refnum<visa-resource-name>)  [unwired: 1 out]
          }
          frame #2 {
            # "go back to start"
            n1944 = call "Set Stage Position.vi"("Position"=w2778, "error in"=w2779, "VISA resource name in"=w2780) -> ()  [unwired: 3 out]
          }
          frame #3 {
            # "stop saving"
            n1945 = local write "Stop Saving"(TRUE ("Stop Saving")) -> ()
            n1946 = local write "Stage Moving"(FALSE ("Stage Moving")) -> ()
          }
        }
      }
      event "Move to Position 1", "Move to Position 2", "Move to Position 3", "Move to Position 4", "Move to Position 5", "Lower Ch. Cap.": Value Change {
        n1947 = event-data() -> ()  [unwired: 1 in, 5 out]
        n1948 = Or(x="Move to Position 5", y="Lower Ch. Cap.") -> (x .or. y?=w2786:bool)
        n1949 = Build Array("Move to Position 1", "Move to Position 2", "Move to Position 3", "Move to Position 4", w2786) -> (w2789:bool[])
        n1950 = Boolean Array To Number(Boolean array=w2789) -> (number=w2788:u32)
        n1951 = Logarithm Base 2(1:w2788) -> (0:w2787:dbl)
        n1952 = flat-sequence {
          tunnel: w2787 -> [w2798]
          tunnel: w2784 -> [w2796]
          tunnel: w2783 -> [w2795]
          frame #0 {
            n1953 = local read "Saved Stage Positions"() -> (w2806:dbl[][])
            n1954 = Array Subset(array=w2806, index (row)=w2798, length (row)=1 ("length"), index (col)=1 ("index"), length (col)=3 ("length")) -> (w2803:dbl[][])
            n1955 = Reshape Array(w2803, 3 ("dimension size")) -> (w2801:dbl[])
            n1956 = Array To Cluster(array=w2801) -> (cluster=w2800:cluster{"[0]":dbl, "[1]":dbl, "[2]":dbl})
            n1957 = call "Set Stage Position.vi"("Position"=w2800, "error in"=w2795, "VISA resource name in"=w2796) -> ("error out"=w2799:errorcluster)  [unwired: 2 out]
            n1958 = local write "Stage Moving"(TRUE ("Stage Moving")) -> ()
            n1959 = local write "Stage Control Serial Error"(w2799) -> ()
          }
          frame #1 {
            n1960 = local write "Stage Moving"(FALSE ("Stage Moving")) -> ()
            n1961 = call <vilib>:"Beep.vi"() -> ()  [unwired: 3 in, 9 out]
          }
        }
      }
      event "Got ADig bead": Value Change {
        n1962 = event-data() -> ()  [unwired: 1 in, 5 out]
        n1963 = flat-sequence {
          frame #0 {
            n1964 = local read "Cap 1 Samp Flow ON"() -> (w2810:bool)
            n1965 = case shown="True" w2810 {
              frame False {
              }
              frame True {
